vi "Create AES Key.vi"() -> ()   [LabVIEW 2021, in "dotNET Crypto Key Management.lvlib"]
uses:
  Key Management/dotNET Crypto Key Management.lvlib
  Key Management/CNG Key Info.ctl
  System.Core
panel:
  out "error out":errorcluster
  out "Export":u8[](array[numeric])
  out "Array":errorcluster[](array[cluster])
  in  "Key Length (256)":i32=256
  in  "Export Policy (allow export)":i32(ring)=1 items=["None"=0, "AllowExport"=1, "AllowPlaintextExport"=2, "AllowArchiving"=4, "AllowPlaintextArchiving"=8]
  in  "Key Usage (all usages)":i32(ring)=16777215 items=["None"=0, "Decryption"=1, "Signing"=2, "KeyAgreement"=4, "AllUsages"=16777215]
  out "Private Key (Graph)":u8[](graph)
  out "Public Key (Graph)":u8[](graph)
  out "Public Key":u8[](array[numeric])
  out "Private Key":u8[](array[numeric])
  out "Key Information":T1
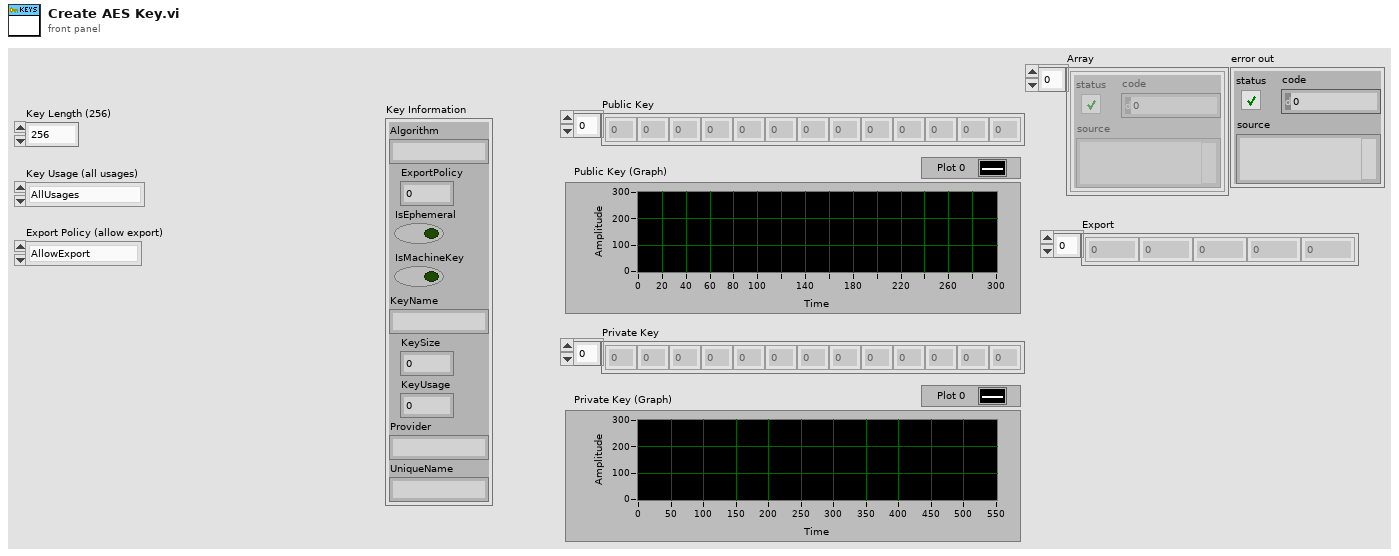
[diagram p1: front panel]
types:
  T1 = typedef "dotNET Crypto Key Management.lvlib/CNG Key Info.ctl" = cluster{"Algorithm":string, "ExportPolicy":i32, "IsEphemeral":bool, "IsMachineKey":bool, "KeyName":string, "KeySize":i32, "KeyUsage":i32, "Provider":string, "UniqueName":string}
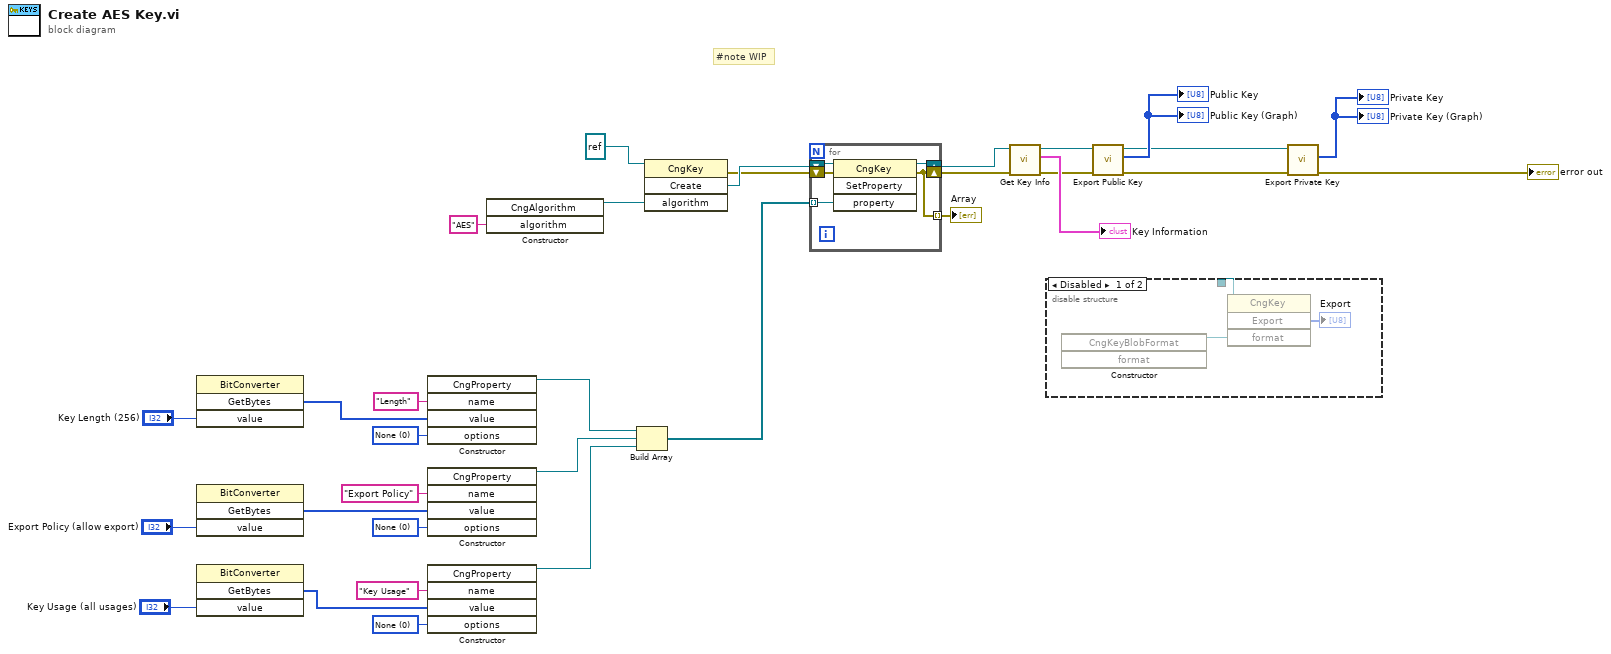
[diagram p0: block diagram]
diagram:
  w21 = 0 items=["None"=0, "CustomProperty"=1073741824, "Persist"=-2147483648] ("options")
  w24 = 0 items=["None"=0, "CustomProperty"=1073741824, "Persist"=-2147483648] ("options")
  w25 = 0 items=["None"=0, "CustomProperty"=1073741824, "Persist"=-2147483648] ("options")
  # "#note WIP"
  n1 = invoke class="BitConverter" method="GetBytes"("value"="Key Length (256)") -> ("GetBytes"=w18:u8[])  [unwired: 3 in, 3 out]
  n2 = invoke class="BitConverter" method="GetBytes"("value"="Export Policy (allow export)") -> ("GetBytes"=w17:u8[])  [unwired: 3 in, 3 out]
  n3 = invoke class="BitConverter" method="GetBytes"("value"="Key Usage (all usages)") -> ("GetBytes"=w16:u8[])  [unwired: 3 in, 3 out]
  n4 = constructor class="CngProperty"("name"="Length", "value"=w18, "options"=w25) -> (reference out=w1:refnum<k24>)  [unwired: 3 in, 5 out]
  n5 = constructor class="CngProperty"("name"="Export Policy", "value"=w17, "options"=w24) -> (reference out=w20:refnum<k24>)  [unwired: 3 in, 5 out]
  n6 = constructor class="CngProperty"("name"="Key Usage", "value"=w16, "options"=w21) -> (reference out=w19:refnum<k24>)  [unwired: 3 in, 5 out]
  n7 = constructor class="CngAlgorithm"("algorithm"="AES") -> (reference out=w30:refnum<k24>)  [unwired: 3 in, 3 out]
  n8 = Build Array(w1, w20, w19) -> (w11:refnum<k24>[])
  n9 = invoke class="CngKey" method="Create"(reference=refnum<k24> refnum, "algorithm"=w30) -> (error out=w13:errorcluster, "Create"=w15:refnum<k24>)  [unwired: 2 in, 2 out]
  n10 = for {
    tunnel: w11 -> [w35] mode=indexing
    shift-right: [w34] -> w14
    shift-left: w15 -> [w36]
    tunnel: [w33] -> w7 mode=indexing
    shift-right: [w33] -> w12
    shift-left: w13 -> [w37]
    n11 = invoke class="CngKey" method="SetProperty"(reference=w36, error in=w37, "property"=w35) -> (reference out=w34:refnum<k24>, error out=w33:errorcluster)  [unwired: 1 in, 2 out]
  }
  "Array" <- w7
  n12 = call "Get Key Info.vi"("error in (no error)"=w12, "CngKey in"=w14) -> ("error out"=w6:errorcluster, "Key Information"=→"Key Information":T1, "CngKey out"=w5:refnum<k24>)  [unwired: 7 in]
  n13 = disable-structure shown="Disabled" {
    disable-tunnel: _ -> [w40 _]
    frame Disabled {
      n14 = constructor class="CngKeyBlobFormat"() -> (reference out=w38:refnum<k24>)  [unwired: 4 in, 3 out]
      n15 = invoke class="CngKey" method="Export"(reference=w40, "format"=w38) -> ("Export"=→"Export":u8[])  [unwired: 2 in, 3 out]
    }
    frame Enabled {
    }
  }
  n16 = call "Export Public Key.vi"("error in (no error)"=w6, "CngKey ref in"=w5) -> ("error out"=w2:errorcluster, "Public Key"=→"Public Key" →"Public Key (Graph)":u8[], "CngKey ref out"=w4:refnum<k24>)  [unwired: 7 in]
  n17 = call "Export Private Key.vi"("error in (no error)"=w2, "CngKey ref in"=w4) -> ("error out"=→"error out":errorcluster, "Private Key"=→"Private Key" →"Private Key (Graph)":u8[])  [unwired: 7 in, 1 out]
